vi "Smooth Transition to Sweep Hold.vi"(6 "Return to 0?":bool, 7 "0 to +(T)\n0 to - (F)":bool, 8 "error in (no error)":errorcluster, 10 "Hardware Parameters":T2={"Scan Calibration [G/V]"=0.0, "Modulation Calibration [G/V]"=0.0, "Modulation Phase [deg]"=0.0, "Modulation Frequency [Hz]"=0.0, "Attenuation [dB]"=0, "Input Channel Count"=0, "Time constant"=7, "Sensitivity"=17, "Frequency Output Voltage [V]"=0.0, "Phase Output Voltage [V]"=0.0, "Lock-in Offset Compensation"=FALSE, "RF [GHz]"=0.0, "Q Start"=0.0, "Q End"=0.0, "Balance"=0.0, "Phase Error"=0.0, "AFC Error"=0.0, "AFC"=FALSE, "Magnet Rotation"=FALSE, "Balance Scaling Factor"=1.0, "Phase Error Scaling Factor"=1.0, "AFC Error Scaling Factor"=1.0, "Frequency Counter ID"="", "Sweep Waveform"=enum."Sawtooth", "Q-Factor Scale"=0.0, " Q-Data Scale"=0.0, " Q-Data Offset"=0.0, "Magnet Rotation Slope"=0.0, "Magnet Rotation Offset"=0.0, "Phase Sweep Resolution"=0.0, "Hardware Version Number"="", "Spectrometer ID Number"=0, "Spectrometer Name"="", "Lock in Saturation"=0.0, "Balance Threshold"=0.0, "Phase Error Threshold"=0.0, "AFC Error Threshold"=0.0, "Linear Actuator Length"=0.0, "Lock-in OK?"=FALSE, "Ignore Lock-in Comm. Failure"=FALSE, "Gradient Addresses"=[], "Gradient Calibrations [G/A*mm]"=[], "Gradient Power Supplies"=[], "Lock-in Address"="", "Magnet Type"=enum."RRI", "Camera Names"=[], "Sweep Limit [Gauss]"=0.0, "Modulation Limit [Gauss]"=0.0, "Balance Threshold Exceeded?"=FALSE, "Phase Threshold Exceeded?"=FALSE, "AFC Threshold Exceeded?"=FALSE, "Consecutive Re-tune attempts"=0, "Reverse Sweep Slope [sec]"=0.0, "Reverse Sweep Offset [G]"=0.0, "AFC Field Correction [V/MHz]"=0.0, "Active Gradients (X Y Z)"=[], "SpO2 Calibration [SpO2/V]"=1.0, "Heart Rate Calibration [BPM/V]"=1.0, "Thermocouple Channel"=""} {"Sensitivity" items=["10 us", "20 us", "40 us", "80 us", "160 us", "320 us", "640 us", "5 ms", "10 ms", "20 ms", "50 ms", "100 ms", "200 ms", "500 ms", "1 s", "2 s", "5 s", "10 s", "20 s", "50 s", "100 s", "200 s", "500 s", "1 ks", "2 ks", "5 ks", "10 ks", "20 ks", "50 ks", "100 ks"]; "Time constant" items=["10 us", "20 us", "40 us", "80 us", "160 us", "320 us", "640 us", "5 ms", "10 ms", "20 ms", "50 ms", "100 ms", "200 ms", "500 ms", "1 s", "2 s", "5 s", "10 s", "20 s", "50 s", "100 s", "200 s", "500 s", "1 ks", "2 ks", "5 ks", "10 ks", "20 ks", "50 ks", "100 ks"]}, 11 "Acquisition Parameters":T1={"Magnet Angle [deg]"=0.0, "Magnet Angles [deg]"=[], "DeltaVpp [v]"=0.0, "SEM [v]"=0.0, "DeltaVpp Thresh [v]"=0.0, "SEM Thresh [v]"=0.0, "Adaptive Processing"=FALSE, "Acquire Q"=FALSE, "Acquire Photos"=FALSE, "Adaptive Tuning"=FALSE, "Automated Matching"=FALSE, "X-Gradient [G/mm]"=0.0, "Y-Gradient [G/mm]"=0.0, "Z-Gradient [G/mm]"=0.0, "Central Field [G]"=0.0, "Scan Width [G]"=0.0, "Mod. Amp. [G]"=0.0, "Scan Time [s]"=0.0, "Pre-Scan Delay [ms]"=0, "Measurement Timeout [s]"=0.0, "Electromagnet Main Field [G]"=0.0, "Locked Central Field [G]"=0.0, "Scans Excluded"=0, "Scans Completed"=0, "No. Scans/Set"=0, "No. Scans for SNR"=0, "Field Locked Frequency [GHz]"=0.0, "Auto Set-based Field Center"=FALSE, "Prompt for oxy acquisition updates"=FALSE, "Oxy QA Scan?"=FALSE, "Exclude Bad Data"=FALSE, "Optimizing RF Power"=FALSE, "Gradients on/off"=FALSE, "Running Script"=TRUE, "Opto-Coupler Current [A]"=0.0, "Continuous Sweeping"=FALSE, "Sweep Rise Time [sec]"=0, "Reverse Sweep Central Field [G]"=0.0, "Forward Sweep Central Field [G]"=0.0, "Sweep Calibrated"=FALSE, "Modulation Calibrated"=FALSE, "First CheckCal Scan?"=FALSE, "AFC Field Correction"=FALSE, "OxyQAInit Scan Width [G]"=0.0, "OxyQAInit Mod. Amp. [G]"=0.0, "Scans Completed/Session"=0, "Acquire SpO2"=FALSE, "Acquire Temperature"=FALSE, "Over Mod"=FALSE} {"OxyQAInit Mod. Amp. [G]" min=0.0; "OxyQAInit Scan Width [G]" min=0.0; "Mod. Amp. [G]" min=0.0; "Scan Width [G]" min=0.0; "Central Field [G]" min=0.0; "Measurement Timeout [s]" min=0.0; "Scan Time [s]" min=0.0; "Z-Gradient [G/mm]" min=0.0; "SEM [v]" min=0.0; "DeltaVpp [v]" min=0.0}) -> (0 "error out":errorcluster)   [LabVIEW 2016]
uses:
  Types/Hardware Parameters.ctl
  Types/Acquisition Parameters.ctl
  Das16.llb/FromEng(array).VI
panel:
  # "Gradients"
  # "Field"
  # "Scans and Sets"
  # "Timing"
  # "Adaptive Dosimetric \nData Processing"
  # "Bridge I/O"
  # "Magnet Rotation"
  # "Field Calibration"
  # "Lock In Amplifier"
  # "Spectrometer Information"
  # "DAQ Settings"
  # "Gradient Coils and Field"
  # "X"
  # "Y"
  # "Z"
  # "Q-Measurements"
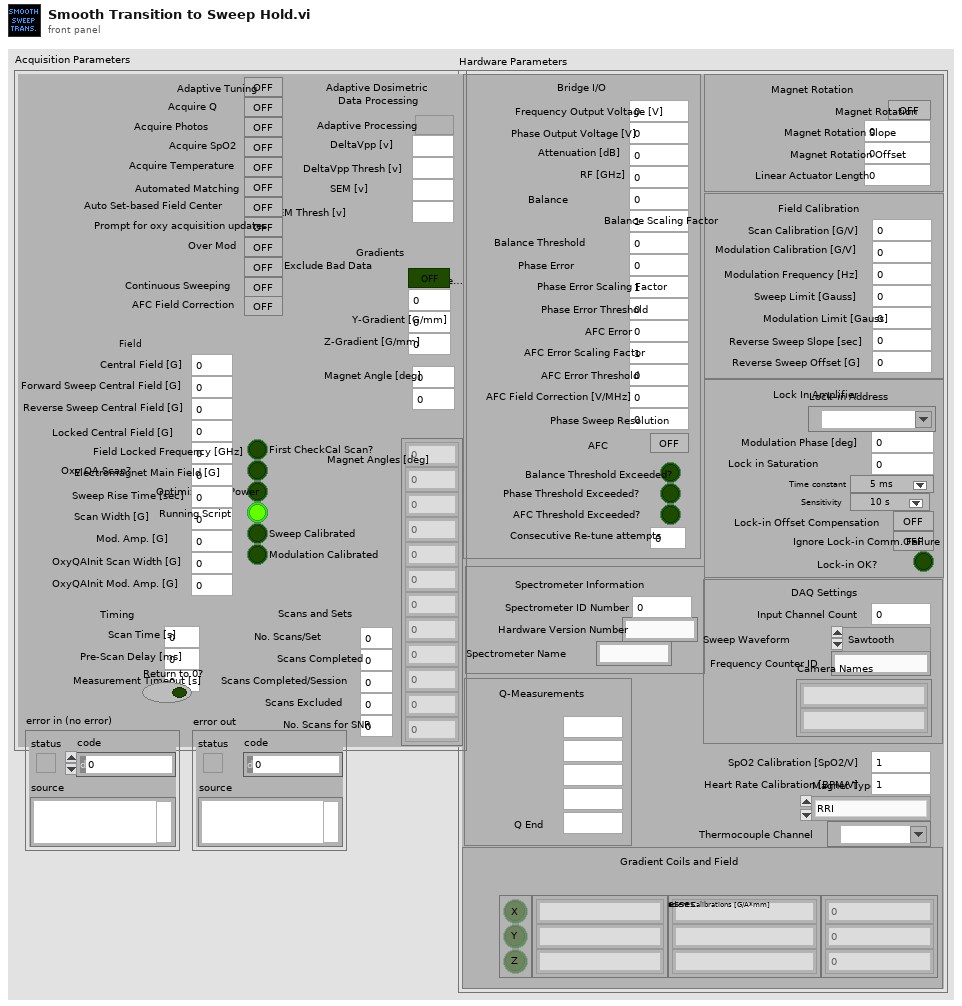
[diagram p1: front panel]
types:
  T1 = typedef "Acquisition Parameters.ctl" = cluster{"Magnet Angle [deg]":dbl, "Magnet Angles [deg]":dbl[], "DeltaVpp [v]":dbl, "SEM [v]":dbl, "DeltaVpp Thresh [v]":dbl, "SEM Thresh [v]":dbl, "Adaptive Processing":bool, "Acquire Q":bool, "Acquire Photos":bool, "Adaptive Tuning":bool, "Automated Matching":bool, "X-Gradient [G/mm]":dbl, "Y-Gradient [G/mm]":dbl, "Z-Gradient [G/mm]":dbl, "Central Field [G]":dbl, "Scan Width [G]":dbl, "Mod. Amp. [G]":dbl, "Scan Time [s]":dbl, "Pre-Scan Delay [ms]":u32, "Measurement Timeout [s]":dbl, "Electromagnet Main Field [G]":dbl, "Locked Central Field [G]":dbl, "Scans Excluded":u32, "Scans Completed":u32, "No. Scans/Set":u32, "No. Scans for SNR":u32, "Field Locked Frequency [GHz]":dbl, "Auto Set-based Field Center":bool, "Prompt for oxy acquisition updates":bool, "Oxy QA Scan?":bool, "Exclude Bad Data":bool, "Optimizing RF Power":bool, "Gradients on/off":bool, "Running Script":bool, "Opto-Coupler Current [A]":dbl, "Continuous Sweeping":bool, "Sweep Rise Time [sec]":u32, "Reverse Sweep Central Field [G]":dbl, "Forward Sweep Central Field [G]":dbl, "Sweep Calibrated":bool, "Modulation Calibrated":bool, "First CheckCal Scan?":bool, "AFC Field Correction":bool, "OxyQAInit Scan Width [G]":dbl, "OxyQAInit Mod. Amp. [G]":dbl, "Scans Completed/Session":u32, "Acquire SpO2":bool, "Acquire Temperature":bool, "Over Mod":bool}
  T2 = typedef "Hardware Parameters.ctl" = cluster{"Scan Calibration [G/V]":dbl, "Modulation Calibration [G/V]":dbl, "Modulation Phase [deg]":dbl, "Modulation Frequency [Hz]":dbl, "Attenuation [dB]":u16, "Input Channel Count":i32, "Time constant":u16, "Sensitivity":u16, "Frequency Output Voltage [V]":dbl, "Phase Output Voltage [V]":dbl, "Lock-in Offset Compensation":bool, "RF [GHz]":dbl, "Q Start":dbl, "Q End":dbl, "Balance":dbl, "Phase Error":dbl, "AFC Error":dbl, "AFC":bool, "Magnet Rotation":bool, "Balance Scaling Factor":dbl, "Phase Error Scaling Factor":dbl, "AFC Error Scaling Factor":dbl, "Frequency Counter ID":string, "Sweep Waveform":enum16{"Sine Wave", "Square Wave", "Sawtooth", "Triangle Wave"}, "Q-Factor Scale":dbl, " Q-Data Scale":dbl, " Q-Data Offset":dbl, "Magnet Rotation Slope":dbl, "Magnet Rotation Offset":dbl, "Phase Sweep Resolution":dbl, "Hardware Version Number":string, "Spectrometer ID Number":i32, "Spectrometer Name":string, "Lock in Saturation":dbl, "Balance Threshold":dbl, "Phase Error Threshold":dbl, "AFC Error Threshold":dbl, "Linear Actuator Length":dbl, "Lock-in OK?":bool, "Ignore Lock-in Comm. Failure":bool, "Gradient Addresses":string[], "Gradient Calibrations [G/A*mm]":dbl[], "Gradient Power Supplies":string[], "Lock-in Address":refnum<visa-resource-name>, "Magnet Type":enum16{"RRI", "BARDA", "Whole Body Permanent", "RRI Electromagnet"}, "Camera Names":string[], "Sweep Limit [Gauss]":dbl, "Modulation Limit [Gauss]":dbl, "Balance Threshold Exceeded?":bool, "Phase Threshold Exceeded?":bool, "AFC Threshold Exceeded?":bool, "Consecutive Re-tune attempts":i32, "Reverse Sweep Slope [sec]":dbl, "Reverse Sweep Offset [G]":dbl, "AFC Field Correction [V/MHz]":dbl, "Active Gradients (X Y Z)":bool[], "SpO2 Calibration [SpO2/V]":dbl, "Heart Rate Calibration [BPM/V]":dbl, "Thermocouple Channel":tag}
  T3 = cluster{"IntnlBoardNum":i32, "Data":i16[], "Size":i32, "IntnlStatus":i32, "IntnlErrCode":i32, "Alias16":u32, "Reserved":i32}
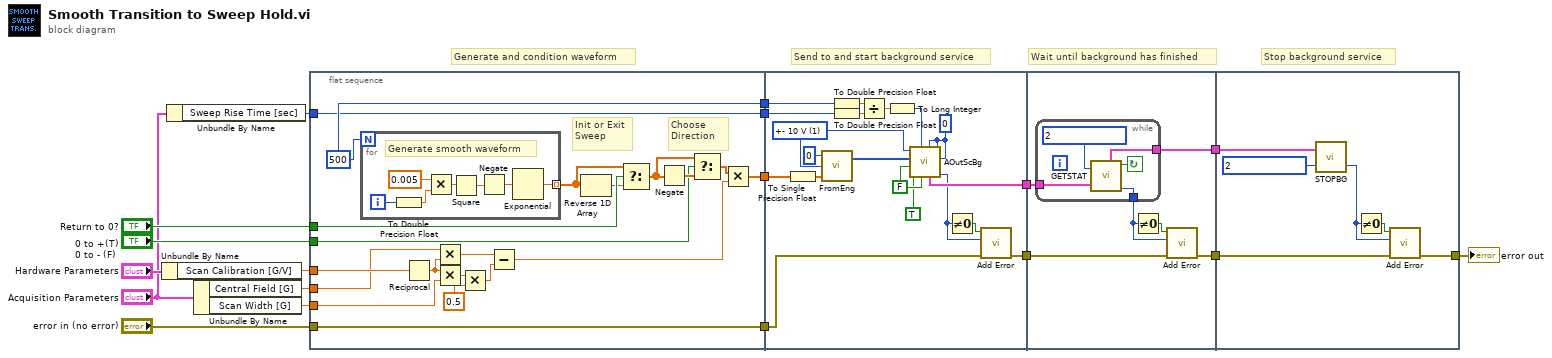
[diagram p0: block diagram]
diagram:
  # "Stop background service"
  # "Wait until background has finished"
  # "Send to and start background service"
  # "Generate and condition waveform"
  n1 = Unbundle By Name("Hardware Parameters") -> ("Scan Calibration [G/V]"=w14:dbl)
  n2 = Unbundle By Name("Acquisition Parameters") -> ("Sweep Rise Time [sec]"=w1:u32)
  n3 = Unbundle By Name("Acquisition Parameters") -> ("Central Field [G]"=w13:dbl, "Scan Width [G]"=w12:dbl)
  n4 = flat-sequence {
    tunnel: [w36] -> w18
    tunnel: [w37] -> w17
    tunnel: w14 -> [w30]
    tunnel: w13 -> [w29]
    tunnel: w12 -> [w28]
    tunnel: "0 to +(T)\n0 to - (F)" -> [w27]
    tunnel: "Return to 0?" -> [w26]
    tunnel: w1 -> [w20]
    tunnel: [w20] -> w8
    tunnel: "error in (no error)" -> [w19]
    tunnel: [w19] -> w6
    tunnel: w18 -> [w58]
    tunnel: [w57] -> w16
    tunnel: w17 -> [w55]
    tunnel: w8 -> [w50]
    tunnel: w6 -> [w47]
    tunnel: [w46] -> w5
    tunnel: w16 -> [w70]
    tunnel: [w69] -> w15
    tunnel: w5 -> [w66]
    tunnel: [w65] -> w4
    tunnel: w15 -> [w81]
    tunnel: w4 -> [w78]
    tunnel: [w76] -> w3
    frame #0 {
      w37 = 500
      # "Choose Direction"
      # "Init or Exit Sweep"
      n5 = for {
        N: w37 -> [_]
        tunnel: [w42] -> w25 mode=indexing
        i -> [w43]
        # "Generate smooth waveform"
        n6 = To Double Precision Float(number=w43) -> (double precision float=w40:dbl)
        n7 = Multiply(x=0.005 ("y"), y=w40) -> (x*y=w45:dbl)
        n8 = Square(x=w45) -> (x^2=w44:dbl)
        n9 = Negate(x=w44) -> (-x=w41:dbl)
        n10 = Exponential(1:w41) -> (0:w42:dbl)
      }
      n11 = Reciprocal(x=w30) -> (1/x=w31:dbl)
      n12 = Multiply(x=w29, y=w31) -> (x*y=w35:dbl)
      n13 = Multiply(x=w31, y=w28) -> (x*y=w32:dbl)
      n14 = Multiply(x=w32, y=0.5) -> (x*y=w34:dbl)
      n15 = Subtract(x=w35, y=w34) -> (x-y=w21:dbl)
      n16 = Reverse 1D Array(array=w25) -> (reversed array=w24:dbl[])
      n17 = Select(t=w25, s=w26, f=w24) -> (s? t:f=w23:dbl[])
      n18 = Negate(x=w23) -> (-x=w38:dbl[])
      n19 = Select(t=w23, s=w27, f=w38) -> (s? t:f=w22:dbl[])
      n20 = Multiply(x=w22, y=w21) -> (x*y=w36:dbl[])
    }
    frame #1 {
      w51 = 0 ("LowChan")
      w63 = FALSE ("Continuous")
      w64 = 1 items=["Not Programmable"=0, "+- 20 V"=27, "+- 10 V"=1, "+- 5 V"=2, "+- 4 V"=28, "+- 2.5 V"=3, "+- 2 V"=29, "+- 1.67 V"=4, "+- 1.25 V"=5, "+- 1 V"=6, "+- .625 V"=7, "+- .5 V"=8, "+- .25 V"=30, "+- .2 V"=31, "+- .1 V"=9, "+- .05 V"=10, "+- .01 V"=11, "+- .005 V"=12, "0 - 10 V"=13, "0 - 5 V"=14, "0 - 4 V"=36, "0 - 2.5 V"=15, "0 - 2 V"=16, "0 - 1.67 V"=17, "0 - 1.25 V"=18, "0 - 1 V"=19, "0 - .5 V"=32, "0 - .25 V"=33, "0 - .2 V"=34, "0 - .1 V"=20, "0 - .02 V"=35, "0 - .01 V"=21, "4 - 20 mA"=22, "2 - 10 mA"=23, "1 - 5 mA"=24, ".5 - 2.5 mA"=25, "0 - 20 mA"=26] ("Range")
      n21 = To Single Precision Float(number=w58) -> (single precision float=w59:sgl[])
      n22 = call-poly "FromEng.VI"("EngUnits"=w59, "Range"=w64, "BoardNum"=u32 0) -> ("DA Data"=w61:u16[])  [unwired: 1 out]
      n23 = To Double Precision Float(number=w55) -> (double precision float=w52:dbl)
      n24 = To Double Precision Float(number=w50) -> (double precision float=w53:dbl)
      n25 = Divide(x=w52, y=w53) -> (x/y=w56:dbl)
      n26 = To Long Integer(number=w56) -> (32bit integer=w54:i32)
      n27 = call "AOutScBg.VI"("BoardNum"=w51, "LowChan"=w51, "HighChan"=w51, "ExtClock"=w63, "Rate"=w54, "Simultaneous"=TRUE, "Continuous"=w63, "DataArray"=w61, "Range"=w64) -> ("ErrCode"=w48:i32, "Context"=w57:T3)  [unwired: 1 out]
      n28 = Not Equal To 0?(x=w48) -> (x != 0?=w49:bool)
      n29 = call "Add Error.vi"("error in (no error)"=w47, "error code (0)"=w48, "error?"=w49) -> ("error out"=w46:errorcluster)  [unwired: 8 in]
    }
    frame #2 {
      n30 = while {
        tunnel: w70 -> [w75]
        tunnel: [w72] -> w69
        tunnel: [w71] -> w67
        stop <- w73 continue-if-true
        n31 = call "GETSTAT.VI"("Function Type"=2, "Context"=w75) -> ("Context"=w72:T3, "Running"=w73:bool, "ErrCode"=w71:i32)  [unwired: 3 out]
      }
      n32 = Not Equal To 0?(x=w67) -> (x != 0?=w68:bool)
      n33 = call "Add Error.vi"("error in (no error)"=w66, "error code (0)"=w67, "error?"=w68) -> ("error out"=w65:errorcluster)  [unwired: 8 in]
    }
    frame #3 {
      n34 = call "STOPBG.VI"("Function Type"=2, "Context"=w81) -> ("ErrorCode"=w77:i32)  [unwired: 1 out]
      n35 = Not Equal To 0?(x=w77) -> (x != 0?=w79:bool)
      n36 = call "Add Error.vi"("error in (no error)"=w78, "error code (0)"=w77, "error?"=w79) -> ("error out"=w76:errorcluster)  [unwired: 8 in]
    }
  }
  "error out" <- w3
